vi "PIO.Windowed Peek.vi"(8 "error in (no error)":errorcluster, 10 "offset":u32 format="%.0x", 11 "GE 5565PIORC in":refnum<class "GE 5565PIORC Old.lvclass">) -> (0 "error out":errorcluster, 2 "value":u32, 3 "GE 5565PIORC out":refnum<class "GE 5565PIORC Old.lvclass">)   [LabVIEW 2016, in "GE 5565PIORC Old.lvclass"]
uses:
  GE 5565PIORC Old.lvclass
  GE 5565PIORC Old.lvclass/GE 5565PIORC Old.ctl
  Registers/Local Configuration.LAS1BA.Local Base Address.Set.vi
  SubVIs/Change Endianness (U32).vi
  Registers/Local Configuration.Get Register Offset.vi
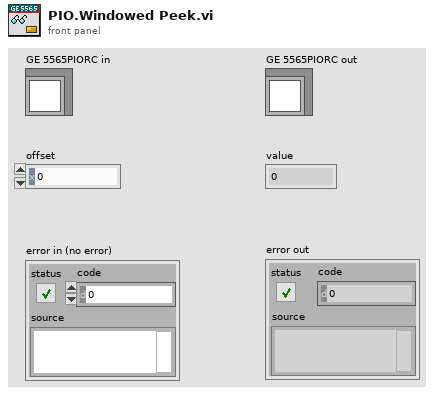
[diagram p1: front panel]
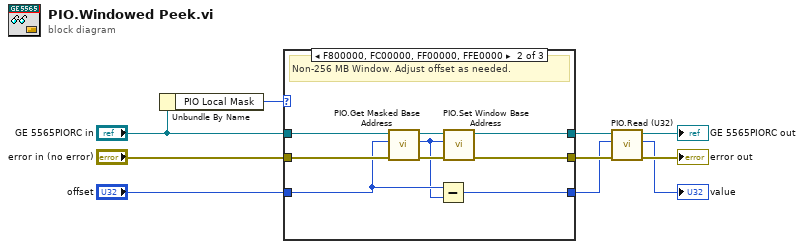
[diagram p0: block diagram]
diagram:
  n1 = Unbundle By Name("GE 5565PIORC in") -> ("PIO Local Mask"=w10:u32)
  n2 = case shown="F800000, FC00000, FF00000, FFE0000" w10 {
    tunnel: "GE 5565PIORC in" -> [w13 w22 w25]
    tunnel: "error in (no error)" -> [w12 w21 w24]
    tunnel: [w13 w16 w25] -> w6
    tunnel: [w12 w15 w24] -> w5
    tunnel: "offset" -> [w11 w20 w23]
    tunnel: [w11 w19 w23] -> w2
    frame 0, Default {
      # "Default case should never be reached."
    }
    frame 260046848, 264241152, 267386880, 268304384 {
      # "Non-256 MB Window. Adjust offset as needed."
      n3 = call "PIO.Get Masked Base Address.vi"("error in (no error)"=w21, "Offset"=w20, "GE 5565PIORC in"=w22) -> ("error out"=w17:errorcluster, "Base Address"=w14:u32, "GE 5565PIORC out"=w18:refnum<class "GE 5565PIORC Old.lvclass">)  [unwired: 6 in]
      n4 = Subtract(x=w20, y=w14) -> (x-y=w19:u32)
      n5 = call "PIO.Set Window Base Address.vi"("error in (no error)"=w17, "Local Base Address"=w14, "GE 5565PIORC in"=w18) -> ("error out"=w15:errorcluster, "GE 5565PIORC out"=w16:refnum<class "GE 5565PIORC Old.lvclass">)  [unwired: 7 in]
    }
    frame 251658240 {
      # "256 MB Window. No adjustment needed."
    }
  }
  n6 = call "PIO.Read (U32).vi"("error in (no error)"=w5, "offset"=w2, "GE 5565PIORC in"=w6) -> ("error out"=→"error out":errorcluster, "value"=→"value":u32, "GE 5565PIORC out"=→"GE 5565PIORC out":refnum<class "GE 5565PIORC Old.lvclass">)  [unwired: 6 in]
